vi "Read Alarm Limits.vi"(8 "error in":errorcluster, 10 "alarm limits in":T1={"Active"=FALSE, "Low Alarm Limit"=variant(dbl 0.0), "Low Warning Limit"=variant(dbl 0.0), "High Warning Limit"=variant(dbl 0.0), "High Alarm Limit"=variant(dbl 0.0), "Low Alarm Severity"=enum."major", "Low Warning Severity"=enum."minor", "High Warning Severity "=enum."minor", "High Alarm Severity"=enum."major", "Hysteresis"=0.0}, 11 "PV Data in":refnum<class "PV Data.lvclass">) -> (0 "error out":errorcluster, 1 "has alarm limits?":bool, 2 "alarm limits out":T1, 3 "PV Data out":refnum<class "PV Data.lvclass">)   [LabVIEW 2020, in "PV Access.lvlib" / "PV Data.lvlib" / "PV Data.lvclass"]
uses:
  PV Data.lvclass
  Write Field (Boolean).vi
  Write Field (Variant).vi
  Write Field (I32).vi
  Write Field (DBL).vi
  Alarm Severity.ctl
  PV Data.lvlib
  Alarm Limits.ctl
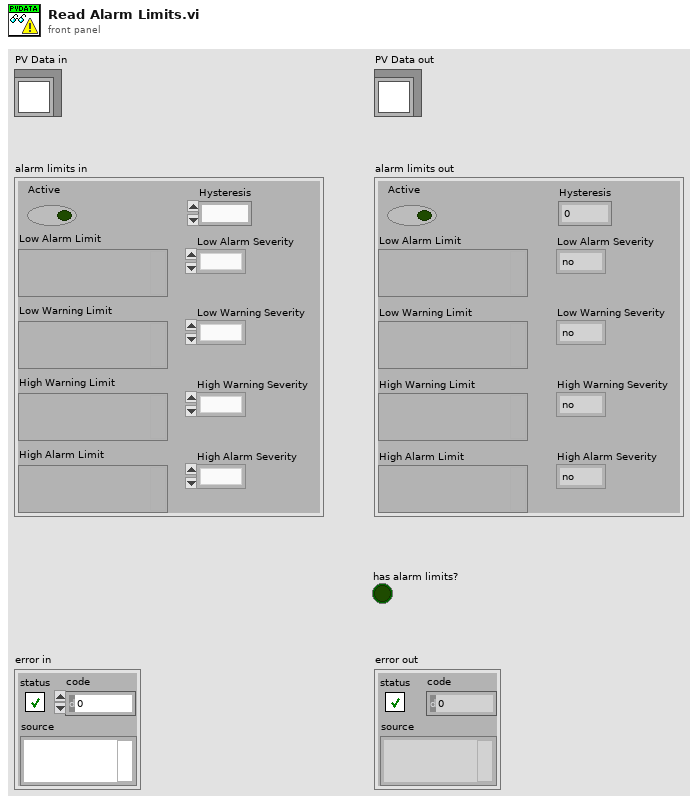
[diagram p1: front panel]
types:
  T1 = typedef "PV Access.lvlib/PV Data.lvlib/Alarm Limits.ctl" = cluster{"Active":bool, "Low Alarm Limit":variant, "Low Warning Limit":variant, "High Warning Limit":variant, "High Alarm Limit":variant, "Low Alarm Severity":T2, "Low Warning Severity":T2, "High Warning Severity ":T2, "High Alarm Severity":T2, "Hysteresis":dbl}
  T2 = typedef "PV Access.lvlib/PV Data.lvlib/Alarm Severity.ctl" = enum32{"no", "minor", "major", "record", "invalid", "undefined", ""}
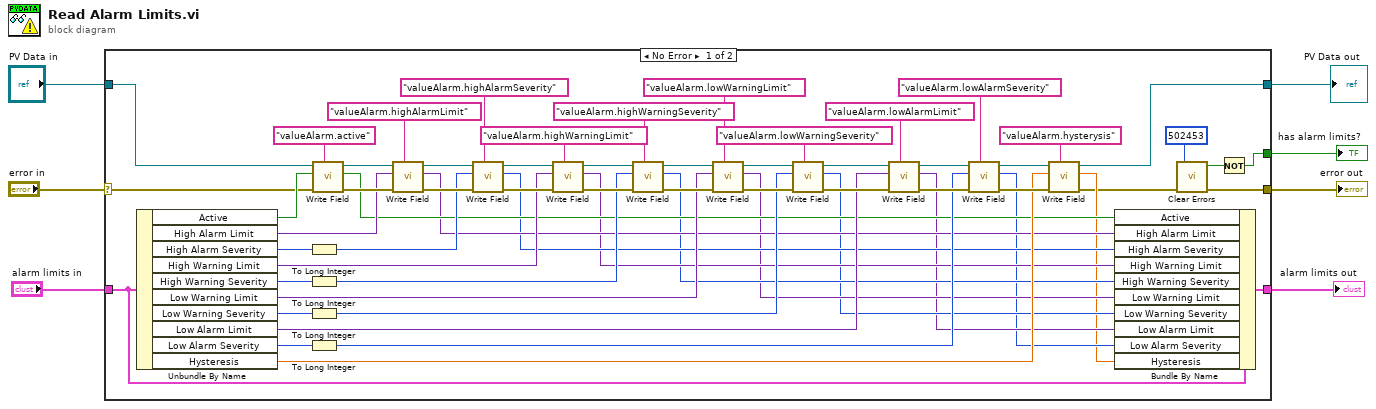
[diagram p0: block diagram]
diagram:
  n1 = case shown="No Error" "error in" {
    selector: "error in" -> [w27 w72]
    tunnel: [w10 w72] -> w5
    tunnel: "PV Data in" -> [w26 w71]
    tunnel: [w25 w71] -> w4
    tunnel: "alarm limits in" -> [w24 w70]
    tunnel: [w13 w70] -> w2
    tunnel: [w8 _] -> w1
    frame No Error {
      n2 = Unbundle By Name(w24) -> ("Active"=w41:bool, "High Alarm Limit"=w40:variant, "High Alarm Severity"=w37:T2, "High Warning Limit"=w33:variant, "High Warning Severity"=w36:T2, "Low Warning Limit"=w31:variant, "Low Warning Severity"=w35:T2, "Low Alarm Limit"=w29:variant, "Low Alarm Severity"=w38:T2, "Hysteresis"=w39:dbl)
      n3 = To Long Integer(number=w37) -> (32bit integer=w34:i32)
      n4 = To Long Integer(number=w36) -> (32bit integer=w32:i32)
      n5 = To Long Integer(number=w35) -> (32bit integer=w30:i32)
      n6 = To Long Integer(number=w38) -> (32bit integer=w28:i32)
      n7 = call-poly "Write Field.vi"("field name"="valueAlarm.active", "error in"=w27, "value"=w41, "PV Data in"=w26) -> ("error out"=w68:errorcluster, "value out"=w23:bool, "PV Data out"=w67:refnum<class "PV Data.lvclass">)  [unwired: 5 in]
      n8 = call-poly "Write Field.vi"("field name"="valueAlarm.highAlarmLimit", "error in (no error)"=w68, "value in"=w40, "PV Data in"=w67) -> ("error out"=w59:errorcluster, "value out"=w22:variant, "PV Data out"=w50:refnum<class "PV Data.lvclass">)  [unwired: 5 in]
      n9 = call-poly "Write Field.vi"("field name"="valueAlarm.highAlarmSeverity", "error in"=w59, "value"=w34, "PV Data in"=w50) -> ("error out"=w60:errorcluster, "value out"=w21:i32, "PV Data out"=w51:refnum<class "PV Data.lvclass">)  [unwired: 5 in]
      n10 = call-poly "Write Field.vi"("field name"="valueAlarm.highWarningLimit", "error in (no error)"=w60, "value in"=w33, "PV Data in"=w51) -> ("error out"=w61:errorcluster, "value out"=w20:variant, "PV Data out"=w52:refnum<class "PV Data.lvclass">)  [unwired: 5 in]
      n11 = call-poly "Write Field.vi"("field name"="valueAlarm.highWarningSeverity", "error in"=w61, "value"=w32, "PV Data in"=w52) -> ("error out"=w62:errorcluster, "value out"=w19:i32, "PV Data out"=w53:refnum<class "PV Data.lvclass">)  [unwired: 5 in]
      n12 = call-poly "Write Field.vi"("field name"="valueAlarm.lowWarningLimit", "error in (no error)"=w62, "value in"=w31, "PV Data in"=w53) -> ("error out"=w63:errorcluster, "value out"=w18:variant, "PV Data out"=w54:refnum<class "PV Data.lvclass">)  [unwired: 5 in]
      n13 = call-poly "Write Field.vi"("field name"="valueAlarm.lowWarningSeverity", "error in"=w63, "value"=w30, "PV Data in"=w54) -> ("error out"=w64:errorcluster, "value out"=w17:i32, "PV Data out"=w55:refnum<class "PV Data.lvclass">)  [unwired: 5 in]
      n14 = call-poly "Write Field.vi"("field name"="valueAlarm.lowAlarmLimit", "error in (no error)"=w64, "value in"=w29, "PV Data in"=w55) -> ("error out"=w65:errorcluster, "value out"=w16:variant, "PV Data out"=w56:refnum<class "PV Data.lvclass">)  [unwired: 5 in]
      n15 = call-poly "Write Field.vi"("field name"="valueAlarm.lowAlarmSeverity", "error in"=w65, "value"=w28, "PV Data in"=w56) -> ("error out"=w58:errorcluster, "value out"=w15:i32, "PV Data out"=w57:refnum<class "PV Data.lvclass">)  [unwired: 5 in]
      n16 = call-poly "Write Field.vi"("field name"="valueAlarm.hysterysis", "error in"=w58, "value"=w39, "PV Data in"=w57) -> ("error out"=w11:errorcluster, "value out"=w14:dbl, "PV Data out"=w25:refnum<class "PV Data.lvclass">)  [unwired: 5 in]
      n17 = Bundle By Name(cluster=w24, "Active"=w23, "High Alarm Limit"=w22, "High Alarm Severity"=w21, "High Warning Limit"=w20, "High Warning Severity"=w19, "Low Warning Limit"=w18, "Low Warning Severity"=w17, "Low Alarm Limit"=w16, "Low Alarm Severity"=w15, "Hysteresis"=w14) -> (w13:T1)
      n18 = call <vilib>:"Clear Errors.vi"("error in (no error)"=w11, "specific error code to clear (0: all)"=502453) -> ("error out"=w10:errorcluster, "specific error cleared?"=w9:bool)  [unwired: 4 in]
      n19 = Not(x=w9) -> (.not. x?=w8:bool)
    }
    frame Error {
    }
  }
  "error out" <- w5
  "PV Data out" <- w4
  "has alarm limits?" <- w1
  "alarm limits out" <- w2
